vi "Create Data Channels.vi"(8 "error in":errorcluster, 11 "Node in":refnum<class "BTSTemplateTest.lvclass">) -> (0 "error out":errorcluster, 3 "Node out":refnum<class "BTSTemplateTest.lvclass">)   [LabVIEW 2023, in "BTSTemplateTest.lvlib" / "BTSTemplateTest.lvclass"]
uses:
  BTSTemplateTest.lvclass
  BTSTemplateTest.lvclass/BTSTemplateTest.ctl
  <vilib>/ADAS Replay HIL/Channels/Tag Wrapper/Polymorphic/Open Producer Tag (Double).vi/45cd6eaa-a1ce-41a4-8aba-62a49d103d7e.vi
  <vilib>/ADAS Replay HIL/Channels/Tag Wrapper/Polymorphic/Open Producer Tag (Double).vi/45cd6eaa-a1ce-41a4-8aba-62a49d103d7e.vi/c28b0ead-42ad-4072-80a2-aca7f2bd7ce3.vi
  <vilib>/ADAS Replay HIL/AdasHilServices/AdasHilServices Fill In Error Info Ex.vi
  <vilib>/ADAS Replay HIL/Template Node/Plugin/Template Node/Template Node.lvclass
  <vilib>/BTS Capabilities/Power Limits/Power Limits.lvclass
  <vilib>/BTS Capabilities/Power/Power Control.lvclass
  <vilib>/BTS Capabilities/Voltage Limits/Voltage Limits.lvclass
  <vilib>/BTS Capabilities/Voltage/Voltage Control.lvclass
  <vilib>/BTS Capabilities/Control Mode/Control Mode.lvclass
  <vilib>/BTS Capabilities/Current/Current Control.lvclass
  <vilib>/BTS Capabilities/Current Limits/Current Limits.lvclass
  <vilib>/BTS Capabilities/Cycler/Cycler.lvclass
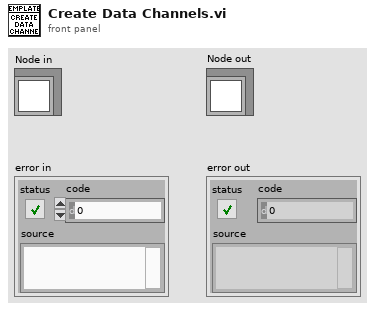
[diagram p1: front panel]
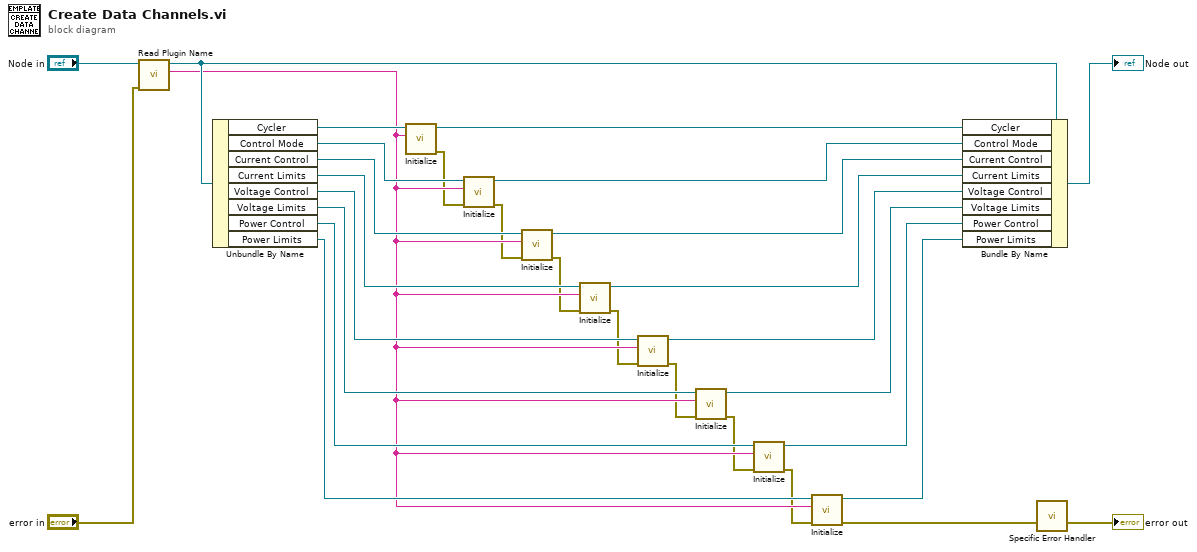
[diagram p0: block diagram]
diagram:
  n1 = call <vilib>:"Read Plugin Name.vi"("error in"="error in", "Template Node in"="Node in") -> ("Plugin Name"=w9:string, "Template Node out"=w25:refnum<class "BTSTemplateTest.lvclass">)  [unwired: 7 in, 1 out]
  n2 = Unbundle By Name(w25) -> ("Cycler"=w27:refnum<class "Cycler.lvclass">, "Control Mode"=w23:refnum<class "Control Mode.lvclass">, "Current Control"=w21:refnum<class "Current Control.lvclass">, "Current Limits"=w20:refnum<class "Current Limits.lvclass">, "Voltage Control"=w16:refnum<class "Voltage Control.lvclass">, "Voltage Limits"=w17:refnum<class "Voltage Limits.lvclass">, "Power Control"=w18:refnum<class "Power Control.lvclass">, "Power Limits"=w19:refnum<class "Power Limits.lvclass">)
  n3 = call-dynamic "Initialize.vi"("Plugin Name"=w9, "Cycler in"=w27) -> ("error out"=w8:errorcluster, "Cycler out"=w26:refnum<class "Cycler.lvclass">)  [unwired: 8 in]
  n4 = call-dynamic "Initialize.vi"("error in"=w8, "Plugin Name"=w9, "Control Mode in"=w23) -> ("error out"=w7:errorcluster, "Control Mode out"=w22:refnum<class "Control Mode.lvclass">)  [unwired: 7 in]
  n5 = call-dynamic "Initialize.vi"("error in"=w7, "Plugin Name"=w9, "Current Control in"=w21) -> ("error out"=w6:errorcluster, "Current Control out"=w15:refnum<class "Current Control.lvclass">)  [unwired: 7 in]
  n6 = call-dynamic "Initialize.vi"("error in"=w6, "Plugin Name"=w9, "Current Limits in"=w20) -> ("error out"=w5:errorcluster, "Current Limits out"=w10:refnum<class "Current Limits.lvclass">)  [unwired: 7 in]
  n7 = call-dynamic "Initialize.vi"("error in"=w5, "Plugin Name"=w9, "Voltage Control in"=w16) -> ("error out"=w4:errorcluster, "Voltage Control out"=w11:refnum<class "Voltage Control.lvclass">)  [unwired: 7 in]
  n8 = call-dynamic "Initialize.vi"("error in"=w4, "Plugin Name"=w9, "Voltage Limits in"=w17) -> ("error out"=w3:errorcluster, "Voltage Limits out"=w12:refnum<class "Voltage Limits.lvclass">)  [unwired: 7 in]
  n9 = call-dynamic "Initialize.vi"("error in"=w3, "Plugin Name"=w9, "Power Control in"=w18) -> ("error out"=w2:errorcluster, "Power Control out"=w13:refnum<class "Power Control.lvclass">)  [unwired: 7 in]
  n10 = call-dynamic "Initialize.vi"("error in"=w2, "Plugin Name"=w9, "Power Limits in"=w19) -> ("error out"=w1:errorcluster, "Power Limits out"=w14:refnum<class "Power Limits.lvclass">)  [unwired: 7 in]
  n11 = Bundle By Name(cluster=w25, "Cycler"=w26, "Control Mode"=w22, "Current Control"=w15, "Current Limits"=w10, "Voltage Control"=w11, "Voltage Limits"=w12, "Power Control"=w13, "Power Limits"=w14) -> (→"Node out":refnum<class "BTSTemplateTest.lvclass">)
  n12 = call "Specific Error Handler"("Error to Check"=w1) -> ("error out"=→"error out":errorcluster)  [unwired: 11 in, 3 out]
